vi "Controller_QueueOperations_FGV.vi"(8 "error in":errorcluster, 10 "Data In":T1={"EntryConsole_Action"=enum."Init", "WashDisplay_Action"=enum."Init", "Controller_Action"=enum."Init", "VehiclePosition_Action"=enum."Init", "Under Body Wash"=FALSE, "Bug Remover"=FALSE, "Pre-Soak"=FALSE, "High Pressure Wash (default)"=FALSE, "Low Pressure Wax"=FALSE, "Spot Free Rinse"=FALSE, "Tire Shine Foam"=FALSE, "Air Dry"=FALSE, "Start"=FALSE, "Current Vehicle Pos"=1, "Wash Step Info"={"Wash States"=enum."Under Body Wash", "Expected Vehicle Pos"=0, "Step duration"=0.0}} {"Wash Step Info"."Step duration" format="%<%H:%M:%S>t"; "Current Vehicle Pos" items=["Entry", "Station 1", "Station 2", "Station 3", "Exit"]}, 11 "Action":T9) -> (0 "error out":errorcluster, 1 "#elements in queue":i32, 2 "elements in queue":T1[](array[typedef]) {"Wash Step Info"."Step duration" format="%<%H:%M:%S>t"; "Current Vehicle Pos" items=["Entry", "Station 1", "Station 2", "Station 3", "Exit"]}, 3 "queue ref":refnum<queue>)   [LabVIEW 2019]
uses:
  #typedef_Queue_enum.ctl
  #typedef_Data_Controller.ctl
  #typedef_EntryConsole_Action_enum.ctl
  #typedef_WashDisplay_Action_enum.ctl
  #typedef_Controller_Action_enum.ctl
  #typedef_VehiclePosition_Action_enum.ctl
  #typedef_VehiclePos_enum.ctl
  #typedef_WashStepInfo.ctl
  #typedef_WashStates.ctl
  #typedef_Data_Cluster.ctl
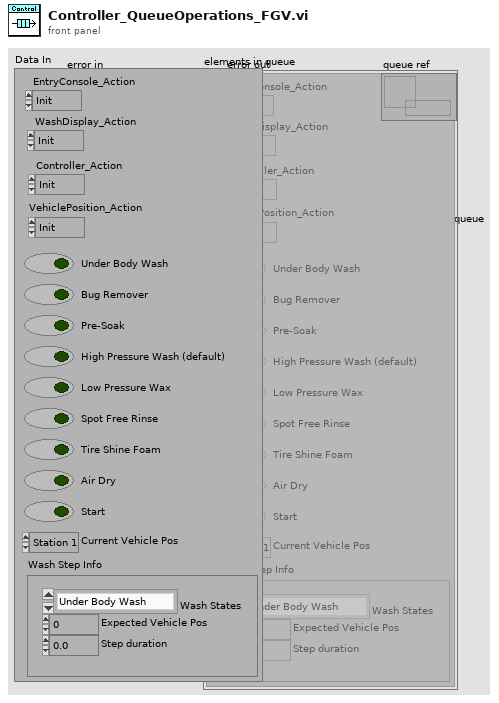
[diagram p1: front panel]
types:
  T1 = typedef "#typedef_Data_Controller.ctl" = cluster{"EntryConsole_Action":T2, "WashDisplay_Action":T3, "Controller_Action":T4, "VehiclePosition_Action":T5, "Under Body Wash":bool, "Bug Remover":bool, "Pre-Soak":bool, "High Pressure Wash (default)":bool, "Low Pressure Wax":bool, "Spot Free Rinse":bool, "Tire Shine Foam":bool, "Air Dry":bool, "Start":bool, "Current Vehicle Pos":T6, "Wash Step Info":T7}
  T2 = typedef "#typedef_EntryConsole_Action_enum.ctl" = enum16{"Init", "ERROR_DEFAULT", "Idle", "Start_Wash_Cycle", "Clear_Console", "Close", "Error_Handler", "Exit"}
  T3 = typedef "#typedef_WashDisplay_Action_enum.ctl" = enum16{"Init", "ERROR_DEFAULT", "Idle", "Update FP", "Close", "Error_Handler", "Exit"}
  T4 = typedef "#typedef_Controller_Action_enum.ctl" = enum16{"ERROR_DEFAULT", "Init", "Read database", "(Idle) Wait for Start", "Start", "Wait for Vehicle Pos", "Wash Step Execution", "Wash Completion", "Wash Exit", "Wash Abort", "Close", "Error Handler", "Exit"}
  T5 = typedef "#typedef_VehiclePosition_Action_enum.ctl" = enum16{"Init", "ERROR_DEFAULT", "Idle", "Close", "Error_Handler", "Exit", "Send Vehicle Pos"}
  T6 = typedef "#typedef_VehiclePos_enum.ctl" = u8
  T7 = typedef "#typedef_WashStepInfo.ctl" = cluster{"Wash States":T8, "Expected Vehicle Pos":i32, "Step duration":dbl}
  T8 = typedef "#typedef_WashStates.ctl" = enum16{"Under Body Wash", "Bug Remover", "Pre-Soak", "High Pressure Wash", "Low Pressure Wax", "Spot Free Rinse", "Tire Shine Foam", "Air Dry"}
  T9 = typedef "#typedef_Queue_enum.ctl" = enum16{"ERROR_default", "Obtain", "Enqueue", "GetStatus", "Flush", "Release"}
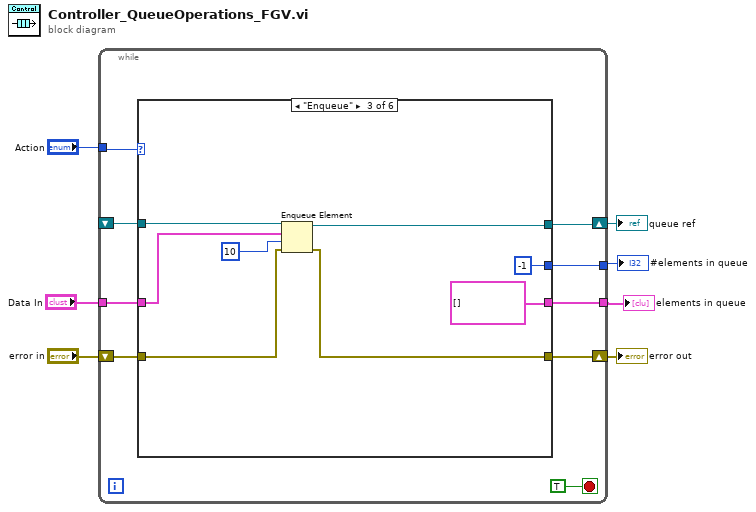
[diagram p0: block diagram]
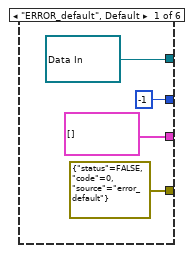
[diagram p2: hidden frame]
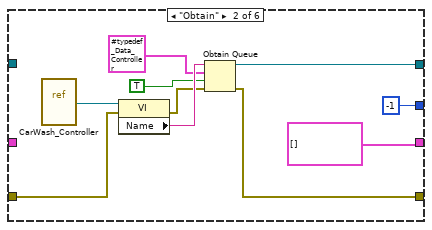
[diagram p3: hidden frame]
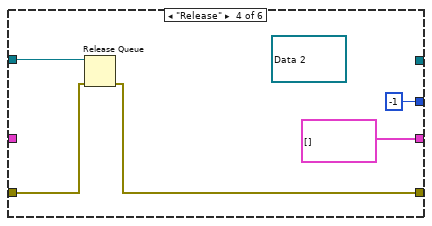
[diagram p4: hidden frame]
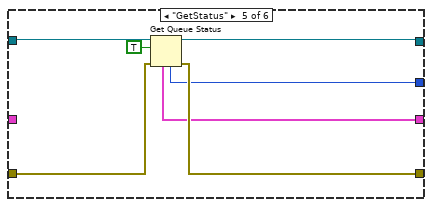
[diagram p5: hidden frame]
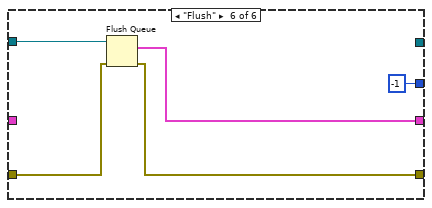
[diagram p6: hidden frame]
diagram:
  n1 = while {
    tunnel: "Action" -> [w15]
    tunnel: "Data In" -> [w13]
    tunnel: [w10] -> w4
    shift-right: [w11] -> w1
    shift-left: _ -> [w9]
    shift-right: [w12] -> w5
    shift-left: "error in" -> [w14]
    tunnel: [w8] -> w2
    stop <- TRUE stop-if-true
    n2 = case shown="\"Enqueue\"" w15 {
      tunnel: w14 -> [_ w30 w37 w42 w47 w54]
      tunnel: w13 -> [_ _ w31 _ _ _]
      tunnel: [errorcluster {"status"=FALSE, "code"=0, "source"="error_default"} ("error out") w27 w36 w41 w48 w53] -> w12
      tunnel: [refnum<queue> refnum ("queue out") w22 w35 _ w49 _] -> w11
      tunnel: [-1 ("# elements in queue") -1 ("#elements in queue") -1 ("#elements in queue") -1 ("# elements in queue") w45 -1 ("# elements in queue")] -> w10
      tunnel: w9 -> [_ _ w38 w43 w50 w55]
      tunnel: [T1[] [] T1[] [] T1[] [] T1[] [] w46 w52] -> w8
      frame "ERROR_default", Default {
      }
      frame "Obtain" {
        n3 = vi-ref "CarWash_Controller.vi"() -> (w24:refnum<vi>)
        n4 = property class="VI"(reference=w24, error in=w30) -> (error out=w28:errorcluster, "Name"=w29:string)  [unwired: 1 out]
        n5 = Obtain Queue(name (unnamed)=w29, element data type=T1 {"EntryConsole_Action"=enum."Init", "WashDisplay_Action"=enum."Init", "Controller_Action"=enum."Init", "VehiclePosition_Action"=enum."Init", "Under Body Wash"=FALSE, "Bug Remover"=FALSE, "Pre-Soak"=FALSE, "High Pressure Wash (default)"=FALSE, "Low Pressure Wax"=FALSE, "Spot Free Rinse"=FALSE, "Tire Shine Foam"=FALSE, "Air Dry"=FALSE, "Start"=FALSE, "Current Vehicle Pos"=1, "Wash Step Info"={"Wash States"=enum."Under Body Wash", "Expected Vehicle Pos"=0, "Step duration"=0.0}} ("Data In"), create if not found? (T)=TRUE, error in (no error)=w28) -> (queue out=w22:refnum<queue>, error out=w27:errorcluster)  [unwired: 1 in, 1 out]
      }
      frame "Enqueue" {
        n6 = Enqueue Element(queue=w38, element=w31, timeout in ms (-1)=10, error in (no error)=w37) -> (queue out=w35:refnum<queue>, error out=w36:errorcluster)  [unwired: 1 out]
      }
      frame "Release" {
        (unwired) refnum<queue> refnum ("queue out")
        n7 = Release Queue(queue=w43, error in (no error)=w42) -> (error out=w41:errorcluster)  [unwired: 1 in, 2 out]
      }
      frame "GetStatus" {
        n8 = Get Queue Status(queue=w50, return elements? (F)=TRUE, error in (no error)=w47) -> (queue out=w49:refnum<queue>, error out=w48:errorcluster, # elements in queue=w45:i32, elements=w46:T1[])  [unwired: 4 out]
      }
      frame "Flush" {
        n9 = Flush Queue(queue=w55, error in (no error)=w54) -> (remaining elements=w52:T1[], error out=w53:errorcluster)  [unwired: 1 out]
      }
    }
  }
  "error out" <- w5
  "#elements in queue" <- w4
  "elements in queue" <- w2
  "queue ref" <- w1
